vi "New Group or Name.vi"(0 "New Group or Experiment.":bool, 3 "Action":T1) -> (7 "New Group or Experiment?":bool)   [LabVIEW 2013]
uses:
  Action Items.ctl
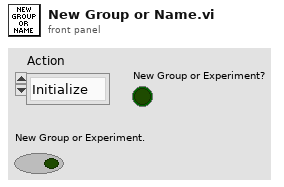
[diagram p1: front panel]
types:
  T1 = typedef "Action Items.ctl" = enum16{"Initialize", "Get", "Set"}
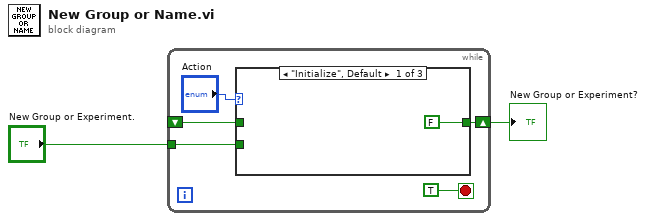
[diagram p0: block diagram]
diagram:
  n1 = while {
    shift-right: [w6] -> w2
    shift-left: _ -> [w5]
    tunnel: "New Group or Experiment." -> [w4]
    stop <- TRUE stop-if-true
    n2 = case shown="\"Initialize\", Default" "Action" {
      tunnel: [FALSE w9 w10] -> w6
      tunnel: w5 -> [_ w9 _]
      tunnel: w4 -> [_ _ w10]
      frame "Initialize", Default {
      }
      frame "Get" {
      }
      frame "Set" {
      }
    }
  }
  "New Group or Experiment?" <- w2
